vi "Simulate Waveguide.vi"(8 "error in (no error)":errorcluster, 9 "Waveguide Cluster":T1={"I+"=0, "I-"=1, "V+"=2, "V-"=3, "Vsg"=4}, 10 "AO":waveform(dbl)[](graph), 11 "Instrument.DAQ in":refnum<class "Instrument.DAQ.lvclass">) -> (0 "error out":errorcluster, 2 "AI":waveform(dbl)[](graph), 3 "Instrument.DAQ out":refnum<class "Instrument.DAQ.lvclass">)   [LabVIEW 2019, in "Instrument.Lockin.lvlib" / "Instrument.DAQ.lvclass"]
uses:
  Instrument.DAQ.lvclass
  d9c89fbe-78e8-46ba-8640-3d5d5975ad94.vi
  Waveguide Model--Cluster.ctl
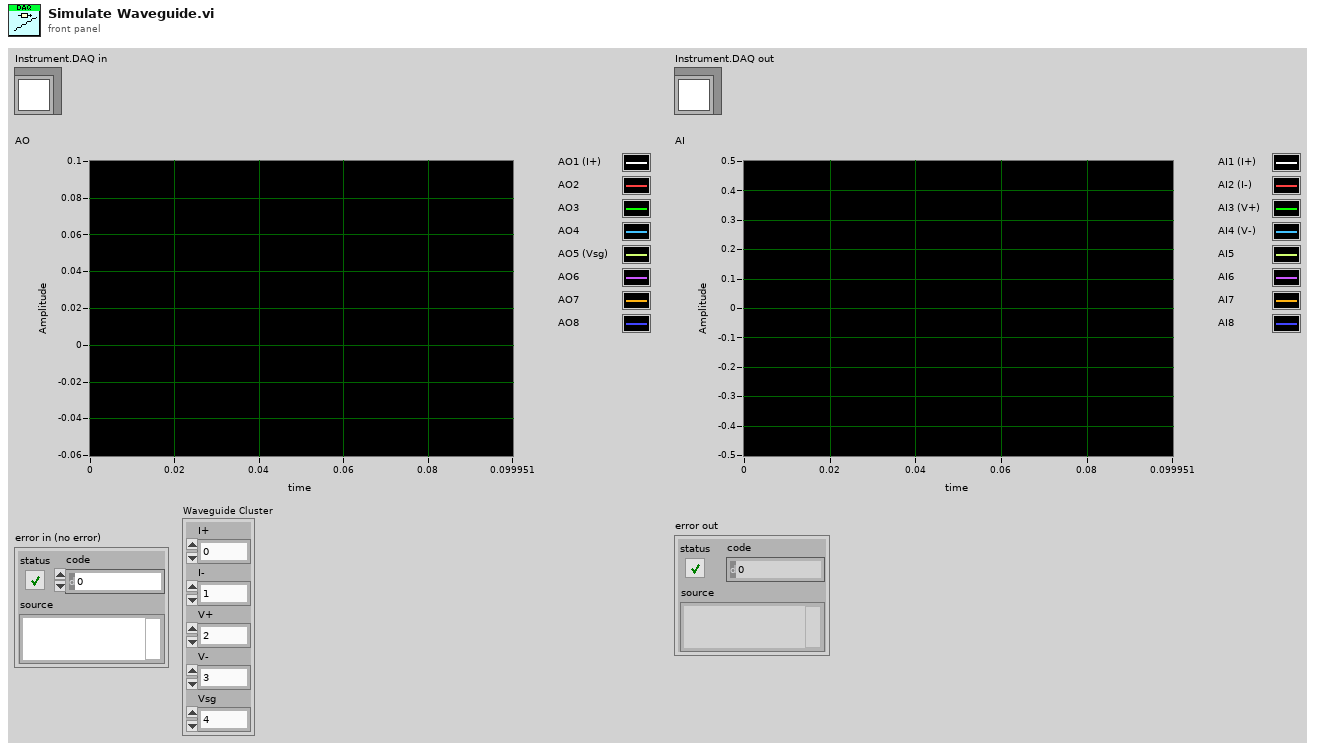
[diagram p1: front panel]
types:
  T1 = typedef "Instrument.Lockin.lvlib/Instrument.DAQ.lvclass/Waveguide Model--Cluster.ctl" = cluster{"I+":i32, "I-":i32, "V+":i32, "V-":i32, "Vsg":i32}
  T2 = typedef "Instrument.Lockin.lvlib/Instrument.DAQ.lvclass/Channel.Gain--Cluster--Array.ctl" = T3[]
  T3 = typedef "Instrument.Lockin.lvlib/Instrument.DAQ.lvclass/Channel.Gain--Cluster.ctl" = cluster{"Channel":string, "Gain":dbl}
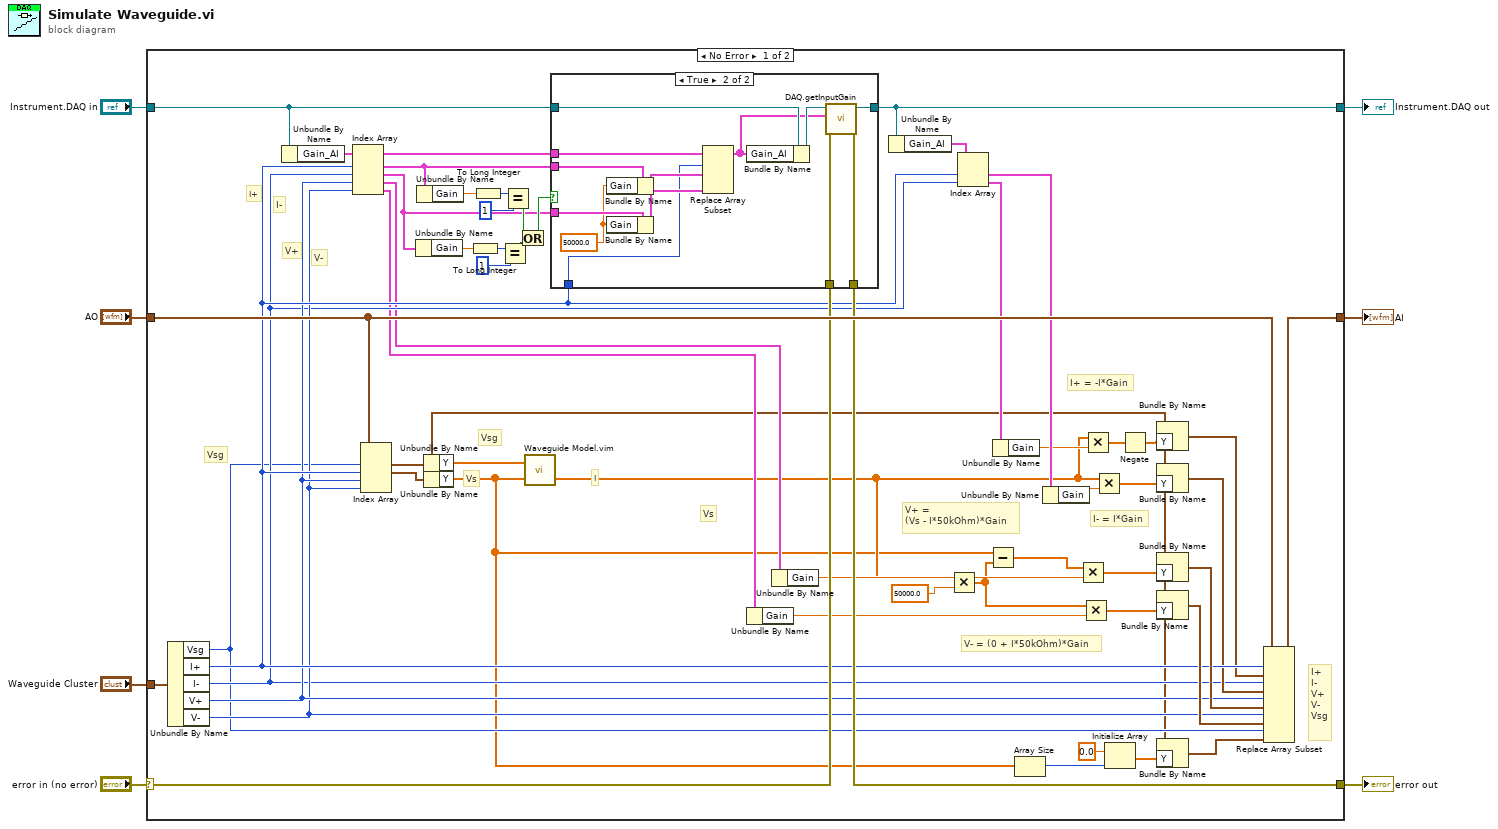
[diagram p0: block diagram]
diagram:
  n1 = case shown="No Error" "error in (no error)" {
    selector: "error in (no error)" -> [w43 w77]
    tunnel: "Waveguide Cluster" -> [w61 _]
    tunnel: [w58 w78] -> w6
    tunnel: [w42 w77] -> w4
    tunnel: [w47 w79] -> w3
    tunnel: "Instrument.DAQ in" -> [w48 w79]
    tunnel: "AO" -> [w59 w78]
    frame No Error {
      # "V- = (0 + I*50kOhm)*Gain"
      # "V+ =\n(Vs - I*50kOhm)*Gain"
      # "I+ = -I*Gain"
      # "I- = I*Gain"
      # "Vsg"
      # "V-"
      # "V+"
      # "Vs"
      # "I-"
      # "I+"
      # "I+\nI-\nV+\nV-\nVsg"
      # "I"
      # "Vs"
      # "Vsg"
      n2 = Unbundle By Name(w61) -> ("Vsg"=w16:i32, "I+"=w40:i32, "I-"=w24:i32, "V+"=w38:i32, "V-"=w28:i32)
      n3 = Unbundle By Name(w48) -> ("Gain_AI"=w52:T2)
      n4 = Index Array(array=w52, index #1=w40, index #2=w24, index #3=w38, index #4=w28) -> (element #1=w51:T3, element #2=w31:T3, element #3=w22:T3, element #4=w23:T3)
      n5 = Index Array(array=w59, index #1=w16, index #2=w40, index #3=w38, index #4=w28) -> (element #1=w12:waveform(dbl), element #2=w57:waveform(dbl))  [unwired: 2 out]
      n6 = Unbundle By Name(w31) -> ("Gain"=w35:dbl)
      n7 = Unbundle By Name(w51) -> ("Gain"=w53:dbl)
      n8 = Unbundle By Name(w12) -> ("Y"=w60:dbl[])
      n9 = Unbundle By Name(w57) -> ("Y"=w8:dbl[])
      n10 = To Long Integer(number=w35) -> (32bit integer=w36:i32)
      n11 = To Long Integer(number=w53) -> (32bit integer=w50:i32)
      n12 = Equal?(x=w36, y=1 ("x")) -> (x = y?=w34:bool)
      n13 = Equal?(x=w50, y=1 ("x")) -> (x = y?=w33:bool)
      n14 = Or(x=w33, y=w34) -> (x .or. y?=w32:bool)
      n15 = call "Waveguide Model.vim"("Vs (V)"=w8, "Vsg (V)"=w60) -> ("I[Vsg] (A)"=w18:dbl[])  [unwired: 1 out]
      n16 = case shown="True" w32 {
        tunnel: w52 -> [_ w76]
        tunnel: w51 -> [_ w75]
        tunnel: w40 -> [_ w65]
        tunnel: w48 -> [w63 w69]
        tunnel: [w63 w74] -> w47
        tunnel: w43 -> [w62 w72]
        tunnel: [w62 w71] -> w42
        tunnel: w31 -> [_ w67]
        frame False {
        }
        frame True {
          w64 = 50000.0
          n17 = Bundle By Name(cluster=w75, "Gain"=w64) -> (w73:T3)
          n18 = Bundle By Name(cluster=w67, "Gain"=w64) -> (w66:T3)
          n19 = Replace Array Subset(array=w76, new element #1=w73, index #1=w65, new element #2=w66) -> (w68:T2)  [unwired: 1 in]
          n20 = Bundle By Name(cluster=w69, "Gain_AI"=w68) -> (w70:refnum<class "Instrument.DAQ.lvclass">)
          n21 = call "DAQ.getInputGain.vi"("error in (no error)"=w72, "Input Gain"=w68, "Instrument.DAQ"=w70) -> ("error out"=w71:errorcluster, "Instrument.DAQ out"=w74:refnum<class "Instrument.DAQ.lvclass">)  [unwired: 7 in]
        }
      }
      n22 = Unbundle By Name(w23) -> ("Gain"=w27:dbl)
      n23 = Unbundle By Name(w22) -> ("Gain"=w41:dbl)
      n24 = Unbundle By Name(w47) -> ("Gain_AI"=w46:T2)
      n25 = Multiply(x=w18, y=50000.0) -> (x*y=w10:dbl[])
      n26 = Index Array(array=w46, index #1=w40, index #2=w24) -> (element #1=w45:T3, element #2=w21:T3)
      n27 = Subtract(x=w8, y=w10) -> (x-y=w29:dbl[])
      n28 = Unbundle By Name(w21) -> ("Gain"=w19:dbl)
      n29 = Array Size(array=w8) -> (size(s)=w14:i32)
      n30 = Unbundle By Name(w45) -> ("Gain"=w44:dbl)
      n31 = Multiply(x=w29, y=w41) -> (x*y=w56:dbl[])
      n32 = Multiply(x=w10, y=w27) -> (x*y=w9:dbl[])
      n33 = Multiply(x=w18, y=w19) -> (x*y=w17:dbl[])
      n34 = Multiply(x=w18, y=w44) -> (x*y=w20:dbl[])
      n35 = Initialize Array(0.0 ("element"), w14) -> (w13:dbl[])
      n36 = Negate(x=w17) -> (-x=w26:dbl[])
      n37 = Bundle By Name(cluster=w12, "Y"=w26) -> (w25:waveform(dbl))
      n38 = Bundle By Name(cluster=w12, "Y"=w20) -> (w39:waveform(dbl))
      n39 = Bundle By Name(cluster=w12, "Y"=w56) -> (w55:waveform(dbl))
      n40 = Bundle By Name(cluster=w12, "Y"=w9) -> (w54:waveform(dbl))
      n41 = Bundle By Name(cluster=w12, "Y"=w13) -> (w11:waveform(dbl))
      n42 = Replace Array Subset(array=w59, new element #1=w25, index #1=w40, new element #2=w39, index #2=w24, new element #3=w55, index #3=w38, new element #4=w54, index #4=w28, new element #5=w11, index #5=w16) -> (w58:waveform(dbl)[])
    }
    frame Error {
    }
  }
  "error out" <- w4
  "Instrument.DAQ out" <- w3
  "AI" <- w6
